vi "LAB3.vi"() -> ()   [LabVIEW 2011]
uses:
  <userlib>/KNR LabVIEW Toolkit/Type Definitions/Port Number (for DC).ctl
  <userlib>/KNR LabVIEW Toolkit/General/KNR Open (Direct Mode).vi
  <userlib>/KNR LabVIEW Toolkit/DC Motor Control/DC Motor Library.lvlib
panel:
  out "sampling time":u32
  out "speed(+-100%)":dbl
  out "e":dbl
  out "current velocity(cm/s)":dbl
  out "Waveform Chart":dbl(graph)
  in  "desired velocity(cm/s)":dbl(slide) scale=-40.0..40.0
  in  "Reverse Encoder?":bool
  in  "Reset Encoder":bool
  out "Position":i32
  in  "Enable Motor":bool
  in  "Port Number":T1=4 items=["Port 1"=4, "Port 2"=5, "Port 3"=6, "Port 4"=7, "Port 5"=8, "Port 6"=9, "Port 7"=10]
  out "error out":errorcluster
  in  "stop":bool
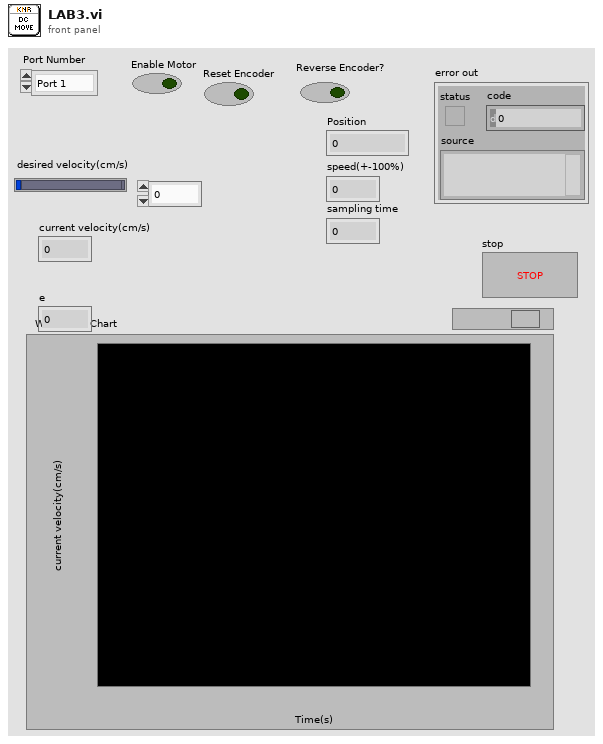
[diagram p1: front panel]
types:
  T1 = typedef "Port Number (for DC).ctl" = u16
  T2 = typedef "KNR Reference.ctl" = cluster{"FPGA Session":refnum<class "FPGA Interface Base.lvclass">, "Port Types":T3[]}
  T3 = typedef "Port Type (API).ctl" = enum8{"Unassigned", "DIO", "DC Motor", "RC Motor", "Ultrasonic", "Analog Input"}
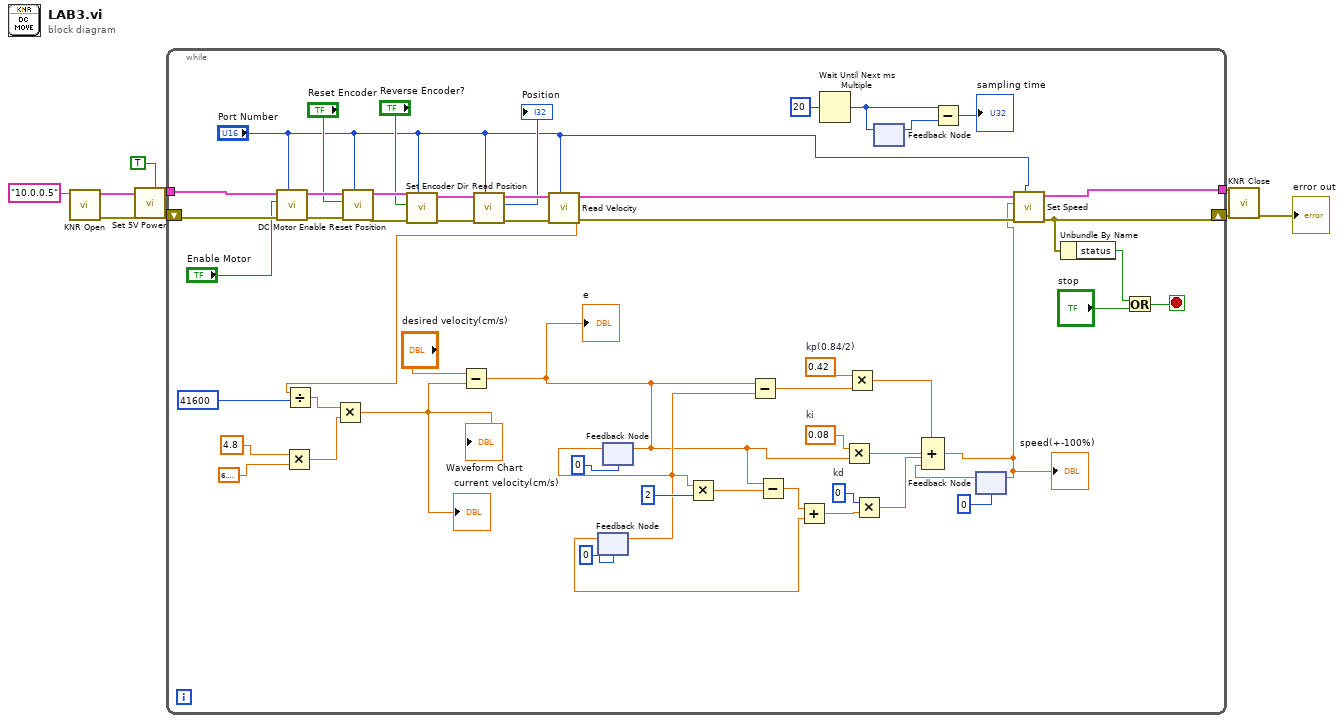
[diagram p0: block diagram]
diagram:
  n1 = call-poly <userlib>:"KNR Open.vi"("IP Address (Default: 10.0.0.5)"="10.0.0.5") -> ("error out"=w8:errorcluster, "KNR Out"=w9:T2)  [unwired: 9 in]
  n2 = call <userlib>:"Set 5V Power.vi"("error in (no error)"=w8, "5V Power"=TRUE, "KNR In"=w9) -> ("error out"=w5:errorcluster, "KNR Out"=w6:T2)  [unwired: 7 in]
  n3 = while {
    tunnel: w6 -> [w59]
    shift-right: [w11] -> w4
    shift-left: w5 -> [w58]
    tunnel: [w35] -> w1
    stop <- w61 stop-if-true
    w22 = 0  # kd
    w30 = 0.08  # ki
    w33 = 0.42  # kp(0.84/2)
    n4 = call <userlib>:"DC Motor Enable.vi"("Port Number"="Port Number", "error in (no error)"=w58, "Enable Motor"="Enable Motor", "KNR In"=w59) -> ("error out"=w53:errorcluster, "KNR Out"=w54:T2)  [unwired: 6 in]
    n5 = Multiply(x=4.8, y=6.283185307179586) -> (x*y=w38:dbl)
    n6 = call <userlib>:"Reset Position.vi"("Port Number"="Port Number", "error in (no error)"=w53, "Reset"="Reset Encoder", "KNR In"=w54) -> ("error out"=w51:errorcluster, "KNR Out"=w52:T2)  [unwired: 6 in]
    n7 = call <userlib>:"Set Encoder Dir.vi"("Port Number"="Port Number", "error in (no error)"=w51, "Reverse?"="Reverse Encoder?", "KNR In"=w52) -> ("error out"=w49:errorcluster, "KNR Out"=w50:T2)  [unwired: 6 in]
    n8 = call <userlib>:"Read Position.vi"("Port Number"="Port Number", "error in (no error)"=w49, "KNR In"=w50) -> ("error out"=w57:errorcluster, "Position"=→"Position":i32, "KNR Out"=w56:T2)  [unwired: 6 in]
    n9 = call <userlib>:"Read Velocity.vi"("Port Number"="Port Number", "error in (no error)"=w57, "KNR In"=w56) -> ("error out"=w47:errorcluster, "Velocity (cts/sec)"=w43:dbl, "KNR Out"=w48:T2)  [unwired: 6 in]
    n10 = Divide(x=w43, y=41600) -> (x/y=w41:dbl)
    n11 = Multiply(x=w41, y=w38) -> (x*y=w36:dbl)
    "Waveform Chart" <- w36
    "current velocity(cm/s)" <- w36
    n12 = Subtract(x="desired velocity(cm/s)", y=w36) -> (x-y=w29:dbl)
    "e" <- w29
    n13 = feedback #1(0 ("kp")) -> (w26:dbl)
    n14 = feedback-in #2(w29) -> ()
    n15 = feedback #2(0 ("kp")) -> (w31:dbl)
    n16 = feedback-in #1(w31) -> ()
    n17 = Multiply(x=w31, y=2 ("kp")) -> (x*y=w28:dbl)
    n18 = Subtract(x=w29, y=w31) -> (x-y=w34:dbl)
    n19 = Subtract(x=w29, y=w28) -> (x-y=w27:dbl)
    n20 = Add(x=w27, y=w26) -> (x+y=w23:dbl)
    n21 = Wait Until Next ms Multiple(millisecond multiple=u32 20) -> (millisecond timer value=w15:u32)
    n22 = Multiply(x=w30, y=w29) -> (x*y=w20:dbl)
    n23 = Multiply(x=w33, y=w34) -> (x*y=w21:dbl)
    n24 = Multiply(x=w22, y=w23) -> (x*y=w19:dbl)
    n25 = feedback #3() -> (w14:u32)  [unwired: 1 in]
    n26 = feedback-in #3(w15) -> ()
    n27 = Subtract(x=w15, y=w14) -> (x-y=→"sampling time":u32)
    n28 = feedback #4(0 ("kp")) -> (w18:dbl)
    n29 = Compound Arithmetic op=ADD(w21, w20, w19, w18) -> (w16:dbl)
    "speed(+-100%)" <- w16
    n30 = feedback-in #4(w16) -> ()
    n31 = call <userlib>:"Set Speed.vi"("Port Number"="Port Number", "error in (no error)"=w47, "Speed (+-100%)"=w16, "KNR In"=w48) -> ("error out"=w11:errorcluster, "KNR Out"=w35:T2)  [unwired: 6 in]
    n32 = Unbundle By Name(w11) -> ("status"=w10:bool)
    n33 = Or(x=w10, y="stop") -> (x .or. y?=w61:bool)
  }
  n34 = call <userlib>:"KNR Close.vi"("error in (no error)"=w4, "KNR In"=w1) -> ("error out"=→"error out":errorcluster)  [unwired: 9 in]
